vi "Untitled 10 (SubVI).vi"(5 "Is Path and Not Empty?":bool, 6 "Number of SPI Buses in":i32, 7 "Replacement VI for SPI Engine":path, 8 "error in (no error)":errorcluster, 9 "VI to which to Add Engines and IO Nodes":path, 10 "LabVIEW Project to Script":path, 11 "Curent Bus Path":path) -> (0 "error out":errorcluster, 3 "Number of SPI Buses out":i32)   [LabVIEW 2014, in "SPI Engine Scripting.lvlib"]
uses:
  SPI Engine Scripting.lvlib
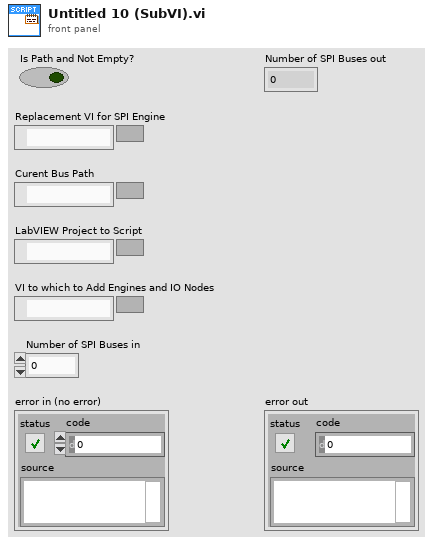
[diagram p1: front panel]
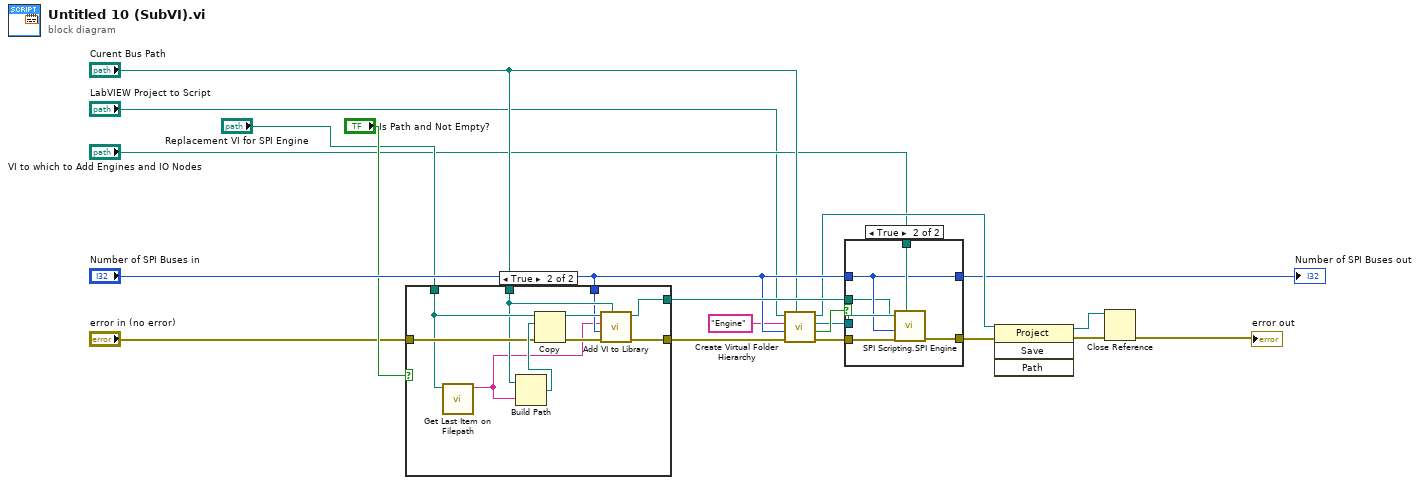
[diagram p0: block diagram]
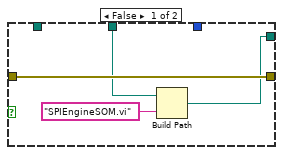
[diagram p2: hidden frame]
diagram:
  n1 = case shown="True" "Is Path and Not Empty?" {
    tunnel: "error in (no error)" -> [w23 w30]
    tunnel: [w23 w29] -> w14
    tunnel: "Replacement VI for SPI Engine" -> [_ w28]
    tunnel: "Curent Bus Path" -> [w21 w27]
    tunnel: "Number of SPI Buses in" -> [_ w26]
    tunnel: [w20 w24] -> w19
    frame False {
      n2 = Build Path(base path=w21, name or relative path="SPIEngineSOM.vi" ("VI to Code Relative Path")) -> (appended path=w20:path)
    }
    frame True {
      n3 = call "Get Last Item on Filepath.vi"("Replacement VI for SPI Engine"=w28) -> ("String"=w25:string)  [unwired: 10 in]
      n4 = Build Path(base path=w27, name or relative path=w25) -> (appended path=w31:path)
      n5 = Copy(8:w30, 10:w31, 11:w28) -> (0:w33:errorcluster, 3:w32:path)  [unwired: 2 in, 1 out]
      n6 = call "Add VI to Library.vi"("Current Bus Path"=w27, "error in"=w33, "Bus Number"=w26, "VI Name"=w25, "Path to new VI"=w32) -> ("error out"=w29:errorcluster, "Path to new IO Node"=w24:path)  [unwired: 5 in]
    }
  }
  n7 = call "Create Virtual Folder Hierarchy.vi"(7:"Curent Bus Path", "error in"=w14, "Bus Number"="Number of SPI Buses in", "Virtual Folder Name"="Engine", "Path to Project"="LabVIEW Project to Script") -> ("error out"=w9:errorcluster, "FPGA Target Found"=w7:bool, "New Virtual Folder"=w6:refnum<vi>, "Project:Open"=w10:refnum<vi>)  [unwired: 3 in]
  n8 = case shown="True" w7 {
    tunnel: "VI to which to Add Engines and IO Nodes" -> [_ w41]
    tunnel: w9 -> [w35 w40]
    tunnel: "Number of SPI Buses in" -> [w34 w37]
    tunnel: [w35 w39] -> w8
    tunnel: w6 -> [_ w38]
    tunnel: [w34 w37] -> w4
    tunnel: w19 -> [_ w36]
    frame False {
    }
    frame True {
      n9 = call "SPI Scripting.SPI Engine.vi"("Path to Place SPI Engine"=w41, "error in"=w40, "Bus Number"=w37, 10:w38, "Path to Engine"=w36) -> ("error out"=w39:errorcluster)  [unwired: 6 in]
    }
  }
  "Number of SPI Buses out" <- w4
  n10 = invoke class="Project" method="Save"(reference=w10, error in=w8) -> (reference out=w12:refnum<vi>, error out=w11:errorcluster)  [unwired: 2 in, 2 out]
  n11 = Close Reference(reference=w12, error in (no error)=w11) -> (error out=→"error out":errorcluster)
